vi "Create.vi"(7 "Direction":T1, 8 "error in (no error)":errorcluster, 9 "Custom Config Data":u8[](array[numeric]), 10 "Name":string, 11 "CIFFIFO in":refnum<class "CIF_NIChn_Fifo_U8.lvclass">) -> (0 "error out":errorcluster, 3 "CIFFIFO out":refnum<class "CIF_NIChn_Fifo_U8.lvclass">)   [LabVIEW 2021, in "CIF_NIChn_Fifo_U8.lvclass"]
uses:
  CIF_NIChn_Fifo_U8.lvclass
  D:/dev/Packages/Channel_Manager/src/CIFChannels/CIFChannels.lvclass
  D:/dev/Packages/Channel_Manager/src/CIF_NIChn/NIChn/CIF_NIChn.lvclass
  CIFChannels/Typedef/Direction.ctl
  <vilib>/CIF Foundation/CIF Utilities/Statistics/I64/Stats_I64_CIF_U.lvclass/Stats_I64_CIF_U.ctl
  CIFChannels/Typedef/Disconnect Behavior.ctl
  CIFChannels/CIFChannels.lvclass/CIFChannels.ctl
  CIF_NIChn_Fifo_U8.lvclass/CIF_NIChn_Fifo_U8.ctl
  CIFChannels/Typedef/Channel State.ctl
  NIChn/CIF_NIChn.lvclass/CIF_NIChn.ctl
  c6f1aac1-fdda-4143-8087-f9e7d57e6170.vi
  05c6e502-0377-480c-a15d-085597602460.vi
  CIFChannels/Accessors/Write Channel State.vi
  NIChn/Accessors/Write CIF Channel.vi
  CIFChannels/Accessors/Write Channel Benchmark.vi
  CIFChannels/Accessors/Write Flatten Benchmark.vi
  CIFChannels/SubVIs/Get Type from Class.vi
  ChannelCommon/Utilities/Unflatten FIFO Config.vi
  CIFChannels/Utilities/Apply Flags.vi
  CIFChannels/Accessors/Write Type.vi
  CIFChannels/Accessors/Write Channel Class.vi
  CIFChannels/Accessors/Write Direction.vi
  CIFChannels/Accessors/Write Tag Disconnect Behavior.vi
  CIFChannels/Accessors/Write Name.vi
  CIFChannels/Accessors/Write Custom Config Data.vi
  <vilib>/CIF Foundation/CIF Channels/CIFChannels/SubVIs/Add Error.vi
  c6f1aac1-fdda-4143-8087-f9e7d57e6170.vi/c28b0ead-42ad-4072-80a2-aca7f2bd7ce3.vi
  <vilib>/CIF Foundation/CIF Channels/CIFChannels/SubVIs/CIFServices Fill In Error Info Ex.vi
  <vilib>/CIF Foundation/CIF Channels/CIFChannels/SubVIs/Get dll Path.vi
  c6f1aac1-fdda-4143-8087-f9e7d57e6170.vi/259f1102-a6f3-45ef-83a9-e8a266e5a7b9.vi
  05c6e502-0377-480c-a15d-085597602460.vi/c28b0ead-42ad-4072-80a2-aca7f2bd7ce3.vi
  <vilib>/CIF Foundation/CIF Utilities/DataTypes/Unflatten U64.vi
  ChannelCommon/Utilities/Expand FIFO Flags.vi
  <vilib>/CIF Foundation/CIF Utilities/Errors/Append Error Location.vi
  <vilib>/Utility/LVClass/Get LV Class Name.vi
  <vilib>/CIF Foundation/CIF Utilities/Statistics/I64/Stats_I64_CIF_U.lvclass
  CIFChannels/CIFChannels.lvclass
  ChannelCommon/ChannelCommon.lvlib
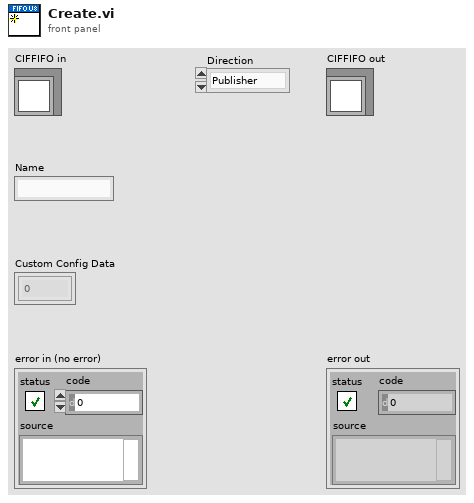
[diagram p1: front panel]
types:
  T1 = typedef "CIFChannels.lvclass/Direction.ctl" = enum16{"Publisher", "Subscriber"}
  T2 = typedef "CIFChannels.lvclass/Disconnect Behavior.ctl" = enum16{"Default value", "Last value", "Error with default"}
  T3 = typedef "CIFChannels.lvclass/Channel State.ctl" = enum16{"Creating", "Disconnected", "Connecting", "Connected", "Destroyed"}
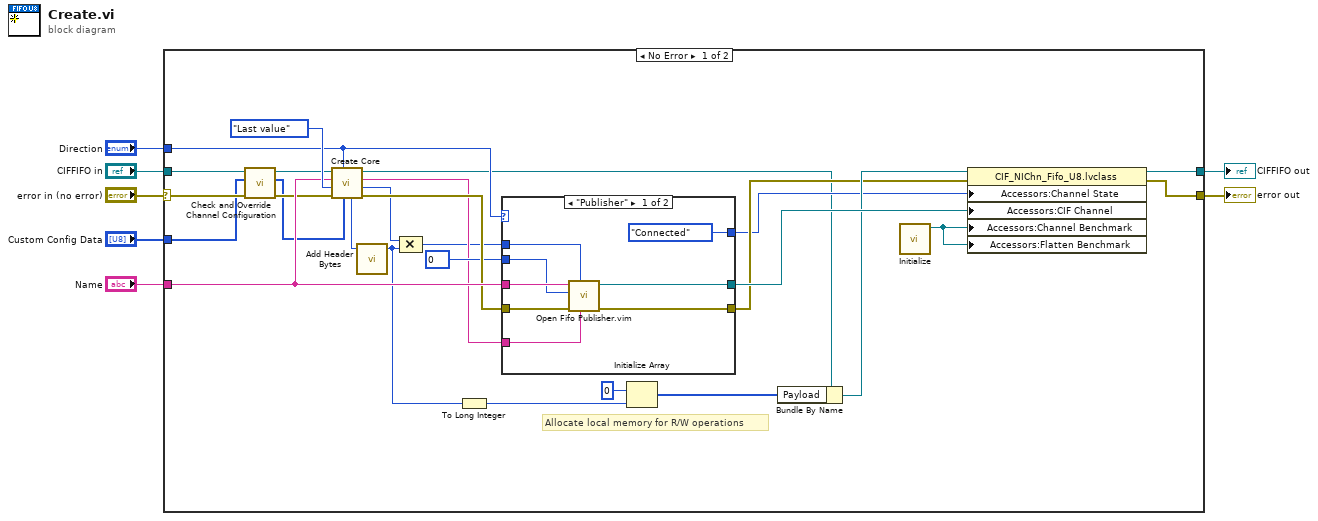
[diagram p0: block diagram]
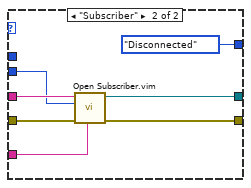
[diagram p2: hidden frame]
diagram:
  n1 = case shown="No Error" "error in (no error)" {
    selector: "error in (no error)" -> [w16 w51]
    tunnel: [w33 w51] -> w6
    tunnel: [w27 w50] -> w4
    tunnel: "CIFFIFO in" -> [w17 w50]
    tunnel: "Name" -> [w32 _]
    tunnel: "Direction" -> [w26 _]
    tunnel: "Custom Config Data" -> [w13 _]
    frame No Error {
      # "Allocate local memory for R/W operations"
      n2 = call-dynamic "Check and Override Channel Configuration.vi"("error in (no error)"=w16, "Custom Config Data in"=w13, "CIFFIFO in"=w17) -> ("error out"=w14:errorcluster, "Custom Config Data out"=w12:u8[], "CIFFIFO out"=w15:refnum<class "CIF_NIChn_Fifo_U8.lvclass">)  [unwired: 6 in]
      n3 = call "Create Core.vi"("Custom Config Data"=w12, "Direction"=w26, "error in (no error)"=w14, "Disconnect Behavior"=Disconnect_Behavior."Last value", "Name"=w32, "CIFChannels in"=w15) -> ("error out"=w31:errorcluster, "Messages"=w11:u64, "Channel Type"=w22:string, "CIFChannels out"=w24:refnum<class "CIF_NIChn_Fifo_U8.lvclass">, "Bytes/Msg"=w10:u64)  [unwired: 1 in]
      n4 = call "Add Header Bytes.vi"("Bytes/Msg"=w10) -> ("Bytes/Msg with header"=w9:u64)  [unwired: 3 in]
      n5 = Compound Arithmetic op=MULTIPLY(w11, w9) -> (w18:u64)
      n6 = To Long Integer(number=w9) -> (32bit integer=w8:i32)
      n7 = case shown="\"Publisher\"" w26 {
        tunnel: w32 -> [w42 w48]
        tunnel: w31 -> [w41 w47]
        tunnel: [w37 w43] -> w30
        tunnel: [w38 w44] -> w28
        tunnel: w22 -> [w40 w46]
        tunnel: [Channel_State."Connected" ("Channel State") Channel_State."Disconnected" ("Channel State")] -> w25
        tunnel: u8 0 -> [w36 w45]
        tunnel: w18 -> [w35 _]
        frame "Publisher" {
          n8 = call "Open Fifo Publisher.vim"("Channel Type Description"=w40, "depth"=w35, "error in"=w41, "Input Type"=w36, "Channel Name"=w42) -> ("error out"=w38:errorcluster, "CIF Channel"=w37:refnum<k21>)  [unwired: 5 in]
        }
        frame "Subscriber" {
          n9 = call "Open Subscriber.vim"("Channel Type Description"=w46, "error in"=w47, "Input Type"=w45, "Channel Name"=w48) -> ("error out"=w44:errorcluster, "CIF Channel"=w43:refnum<k21>)  [unwired: 6 in]
        }
      }
      n10 = Initialize Array(u8 0 ("Numeric"), w8) -> (w20:u8[])
      n11 = Bundle By Name(cluster=w24, "Payload"=w20) -> (w29:refnum<class "CIF_NIChn_Fifo_U8.lvclass">)
      n12 = call <vilib>:"Initialize.vi"() -> ("Stats_I64_CIF_U out"=w19:refnum<class "Stats_I64_CIF_U.lvclass">)  [unwired: 10 in, 1 out]
      n13 = property class="CIF_NIChn_Fifo_U8.lvclass"(reference=w29, error in=w28, "Accessors:Channel State"=w25, "Accessors:CIF Channel"=w30, "Accessors:Channel Benchmark"=w19, "Accessors:Flatten Benchmark"=w19) -> (reference out=w27:refnum<class "CIF_NIChn_Fifo_U8.lvclass">, error out=w33:errorcluster)
    }
    frame Error {
    }
  }
  "error out" <- w6
  "CIFFIFO out" <- w4
